vi "Write Status Cluster.vi"(8 "error in (no error)":errorcluster, 10 "Status Cluster":T1, 11 "HexapodPI in":refnum<class "HexapodPI.lvclass">) -> (0 "error out":errorcluster, 3 "HexapodPI out":refnum<class "HexapodPI.lvclass">)   [LabVIEW 2020, in "HexapodPI.lvclass"]
uses:
  HexapodPI.lvclass
  HexapodPI.lvclass/HexapodPI.ctl
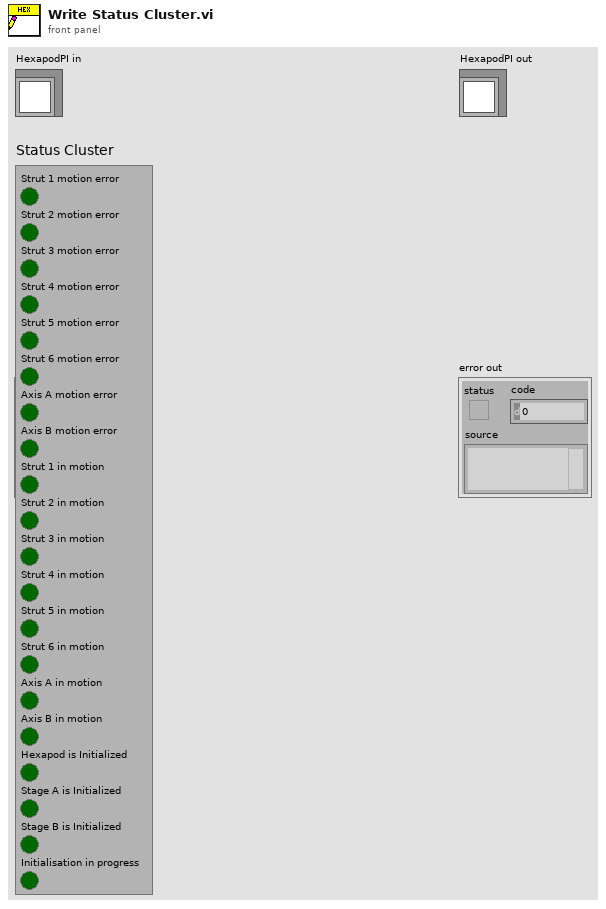
[diagram p1: front panel]
types:
  T1 = cluster{"Strut 1 motion error":bool, "Strut 2 motion error":bool, "Strut 3 motion error":bool, "Strut 4 motion error":bool, "Strut 5 motion error":bool, "Strut 6 motion error":bool, "Axis A motion error":bool, "Axis B motion error":bool, "Strut 1 in motion":bool, "Strut 2 in motion":bool, "Strut 3 in motion":bool, "Strut 4 in motion":bool, "Strut 5 in motion":bool, "Strut 6 in motion":bool, "Axis A in motion":bool, "Axis B in motion":bool, "Hexapod is Initialized":bool, "Stage A is Initialized":bool, "Stage B is Initialized":bool, "Initialisation in progress":bool}
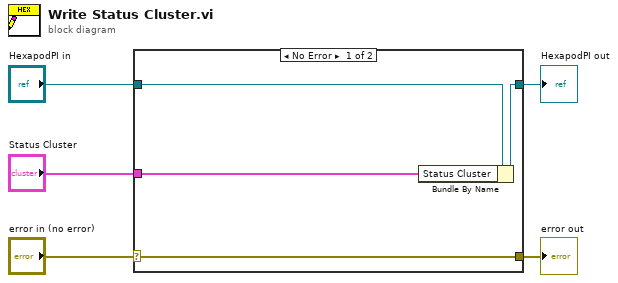
[diagram p0: block diagram]
diagram:
  n1 = case shown="No Error" "error in (no error)" {
    selector: "error in (no error)" -> [w9 w10]
    tunnel: [w9 w10] -> w4
    tunnel: [w7 w11] -> w2
    tunnel: "HexapodPI in" -> [w8 w11]
    tunnel: "Status Cluster" -> [w6 _]
    frame No Error {
      n2 = Bundle By Name(cluster=w8, "Status Cluster"=w6) -> (w7:refnum<class "HexapodPI.lvclass">)
    }
    frame Error {
    }
  }
  "error out" <- w4
  "HexapodPI out" <- w2
